vi "addmul.vi"(1 "Numeric 4":dbl, 2 "Numeric 3":dbl, 3 "Numeric 2":dbl, 4 "Numeric":dbl) -> (0 "Numeric 5":dbl)   [LabVIEW 2021]
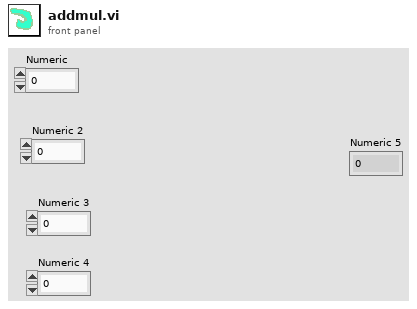
[diagram p1: front panel]
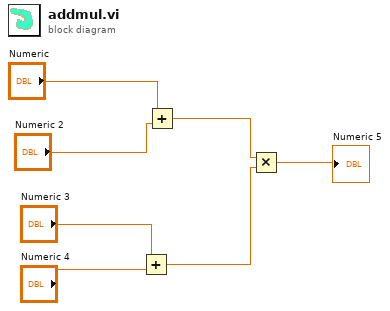
[diagram p0: block diagram]
diagram:
  n1 = Add(x="Numeric 3", y="Numeric 4") -> (x+y=w2:dbl)
  n2 = Add(x="Numeric", y="Numeric 2") -> (x+y=w3:dbl)
  n3 = Multiply(x=w3, y=w2) -> (x*y=→"Numeric 5":dbl)
